vi "Get_ADAM_Ch_names_client.vi"(1 "Channel names set":T1) -> (0 "Ch names":string[](array[string]))   [LabVIEW 2022 SP3]
doc: "This is an example of using features of the VI Server as a client. It shows how you might browse from one or more applications that may be exporting data from one or more data stations. \n\nThe example shows how to query a server for its list of exported VIs, how to get references to the VIs, and how call them with the Call By Reference function."
uses:
  Sub VIs/ADAM Controls/Channel_names.ctl
  Anemometry/Anemometry Sub Vis/Controls/Global_mode.ctl
  Sub VIs/ADAM Controls/Channel_State.ctl
  Anemometry/Anemometry Sub Vis/Globals/Preference_global.vi
panel:
  in  "Server type":refnum<vi>
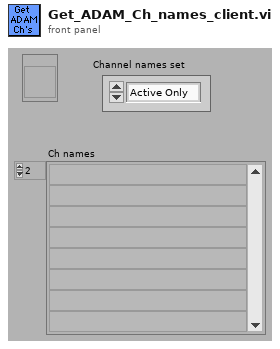
[diagram p1: front panel]
types:
  T1 = typedef "Channel_names.ctl" = enum16{"Active Only", "Active + Off", "All Channels", "Changeable Only", "Always Off", "Always On", "Always Off or On"}
  T2 = typedef "Server_Comms.ctl" = enum16{"Do Not Link To Server", "Server Link Healthy"}
  T3 = typedef "Global_mode.ctl" = enum16{"Read Global", "Load Global From File", "Write Global to File"}
  T4 = typedef "Channel_State.ctl" = enum16{"On", "Off", "Always On", "Always Off"}
  T5 = typedef "Ch_description_ADAM.ctl" = cluster{"Ch Name":string, "Type":T6, "Function":T7, "Ch State":T4, "Calibration type":T8, "A":dbl, "B":dbl, "C":dbl, "D":dbl, "Comments":string, "Address":T9, "String":string, "Duty":u16}
  T6 = typedef "Module_type_ADAM.ctl" = string
  T7 = typedef "Function_ADAM.ctl" = enum16{"Analogue Input", "Digital Input", "Event counter", "Event rate", "Analogue Output", "Digital Output", "Relay Output"}
  T8 = typedef "Calib_type_ADAM.ctl" = string
  T9 = typedef "Address.ctl" = cluster{"Main":i32, "Ch.":i32, "Sub":i32, "Port Name":string}
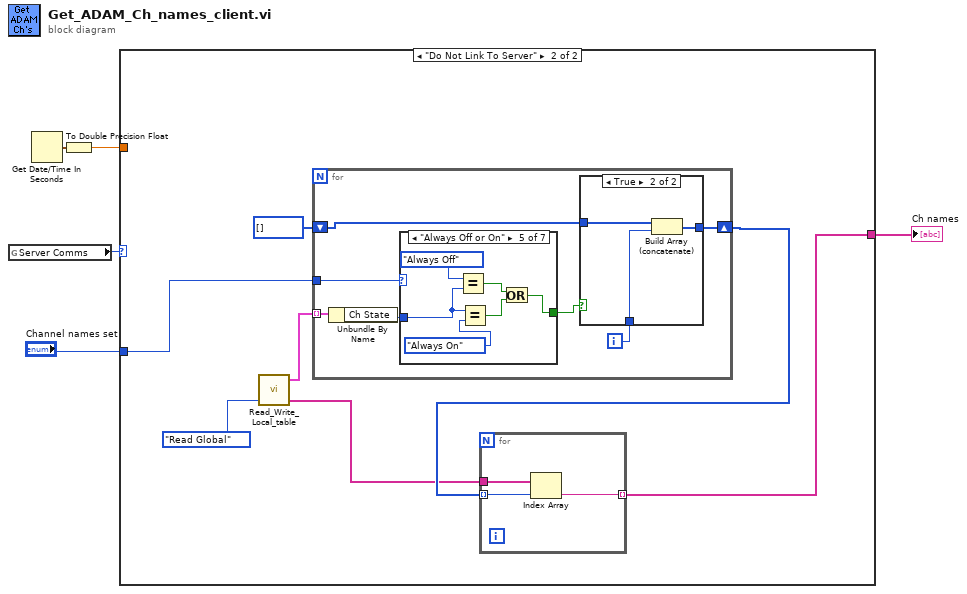
[diagram p0: block diagram]
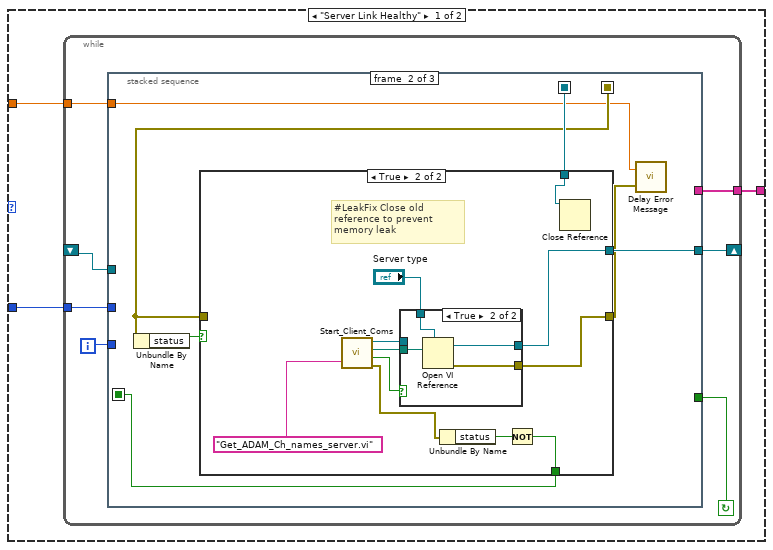
[diagram p2: hidden frame]
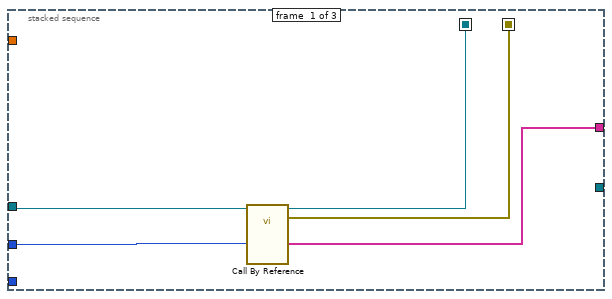
[diagram p3: hidden frame]
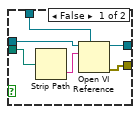
[diagram p5: hidden frame]
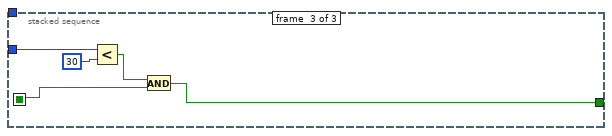
[diagram p6: hidden frame]
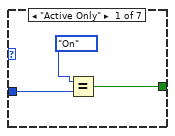
[diagram p8: hidden frame]
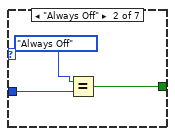
[diagram p9: hidden frame]
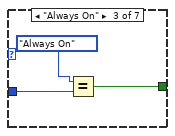
[diagram p10: hidden frame]
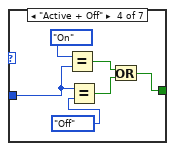
[diagram p11: hidden frame]
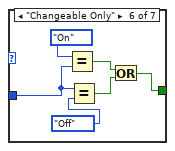
[diagram p12: hidden frame]
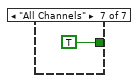
[diagram p13: hidden frame]
diagram:
  n1 = global read "Preference_global.vi" "Server Comms"() -> (w4:T2)
  n2 = Get Date/Time In Seconds() -> (seconds since 1Jan1904=w2:timestamp)
  n3 = To Double Precision Float(number=w2) -> (double precision float=w1:dbl)
  n4 = case shown="\"Do Not Link To Server\"" w4 {
    tunnel: [w8 w57] -> w5
    tunnel: "Channel names set" -> [w7 w61]
    tunnel: w1 -> [w6 _]
    frame "Server Link Healthy" {
      n5 = while {
        tunnel: [w11] -> w8
        shift-left: _ -> [w15]
        shift-right: [w14] -> _
        tunnel: w7 -> [w10]
        tunnel: w6 -> [w9]
        i -> [w13]
        stop <- w12 continue-if-true
        n6 = stacked-sequence {
          seq-local: [w18 _ _] -> [_ w26 _]
          seq-local: [w17 _ _] -> [_ w24 _]
          seq-local: [_ w21 _] -> [_ _ w53]
          tunnel: w15 -> [w20 _ _]
          tunnel: [_ w27 _] -> w14
          tunnel: w13 -> [_ _ w54]
          tunnel: [_ _ w52] -> w12
          tunnel: [w19 _ _] -> w11
          tunnel: w10 -> [w16 _ _]
          tunnel: w9 -> [_ w22 _]
          frame #0 {
            n7 = call-by-ref "?"(reference=w20, "Channel names set"=w16) -> (reference out=w18:refnum<vi>, error out=w17:errorcluster, "Ch names"=w19:string[])  [unwired: 1 in]
          }
          frame #1 {
            n8 = Unbundle By Name(w24) -> ("status"=w25:bool)
            n9 = case shown="True" w25 {
              selector: w25 -> [w28 _]
              tunnel: [w30 w37] -> w27
              tunnel: w26 -> [w30 w34]
              tunnel: [w29 w35] -> w23
              tunnel: w24 -> [w29 _]
              tunnel: [w28 w31] -> w21
              frame False {
              }
              frame True {
                # "#LeakFix Close old reference to prevent memory leak"
                n10 = call "Start_Client_Coms.vi"("VI name to run on server"="Get_ADAM_Ch_names_server.vi") -> ("LabVIEW application reference"=w39:refnum<vi>, "Checked VI name"=w40:path, "Local Call"=w38:bool, "Error cluster"=w32:errorcluster)  [unwired: 1 in]
                n11 = case shown="True" w38 {
                  tunnel: [w44 w51] -> w37
                  tunnel: "Server type" -> [w43 w50]
                  tunnel: w40 -> [w47 w49]
                  tunnel: w39 -> [w42 _]
                  tunnel: [w45 w48] -> w35
                  frame False {
                    n12 = Strip Path(path=w47) -> (name=w46:string)  [unwired: 1 out]
                    n13 = Open VI Reference(type specifier VI Refnum (for type only)=w43, application reference (local)=w42, vi path=w46) -> (vi reference=w44:refnum<vi>, error out=w45:errorcluster)  [unwired: 1 in, 2 out]
                  }
                  frame True {
                    n14 = Open VI Reference(type specifier VI Refnum (for type only)=w50, vi path=w49) -> (vi reference=w51:refnum<vi>, error out=w48:errorcluster)  [unwired: 1 in, 3 out]
                  }
                }
                n15 = Unbundle By Name(w32) -> ("status"=w33:bool)
                n16 = Not(x=w33) -> (.not. x?=w31:bool)
                n17 = Close Reference(reference=w34) -> ()  [unwired: 1 in, 1 out]
              }
            }
            n18 = call "Delay Error Message.vi"("error in (no error)"=w23, "Seconds since 1904"=w22) -> ()  [unwired: 2 in]
          }
          frame #2 {
            n19 = Less?(x=w54, y=30) -> (x < y?=w56:bool)
            n20 = And(x=w56, y=w53) -> (x .and. y?=w52:bool)
          }
        }
      }
    }
    frame "Do Not Link To Server" {
      n21 = call "Read_Write_Local_table.vi"("Mode"=Global_mode."Read Global") -> ("Ch Names"=w58:string[], "Channels Descriptions Out"=w62:T5[])  [unwired: 2 in, 1 out]
      n22 = for {
        tunnel: w62 -> [w73] mode=indexing
        tunnel: w61 -> [w72]
        shift-right: [w68] -> w59
        shift-left: i32[] [] -> [w67]
        i -> [w69]
        n23 = Unbundle By Name(w73) -> ("Ch State"=w71:T4)
        n24 = case shown="\"Always Off or On\"" w72 {
          tunnel: w71 -> [w80 w83 w86 w91 w97 w103 _]
          tunnel: [w78 w81 w84 w87 w93 w99 TRUE] -> w70
          frame "Active Only" {
            n25 = Equal?(x=Channel_State."On" ("Ch State"), y=w80) -> (x = y?=w78:bool)
          }
          frame "Always Off" {
            n26 = Equal?(x=Channel_State."Always Off" ("Ch State"), y=w83) -> (x = y?=w81:bool)
          }
          frame "Always On" {
            n27 = Equal?(x=Channel_State."Always On" ("Ch State"), y=w86) -> (x = y?=w84:bool)
          }
          frame "Active + Off" {
            n28 = Equal?(x=Channel_State."On" ("Ch State"), y=w91) -> (x = y?=w88:bool)
            n29 = Equal?(x=w91, y=Channel_State."Off" ("Ch State")) -> (x = y?=w89:bool)
            n30 = Or(x=w88, y=w89) -> (x .or. y?=w87:bool)
          }
          frame "Always Off or On" {
            n31 = Equal?(x=Channel_State."Always Off" ("Ch State"), y=w97) -> (x = y?=w94:bool)
            n32 = Equal?(x=w97, y=Channel_State."Always On" ("Ch State")) -> (x = y?=w95:bool)
            n33 = Or(x=w94, y=w95) -> (x .or. y?=w93:bool)
          }
          frame "Changeable Only" {
            n34 = Equal?(x=Channel_State."On" ("Ch State"), y=w103) -> (x = y?=w100:bool)
            n35 = Equal?(x=w103, y=Channel_State."Off" ("Ch State")) -> (x = y?=w101:bool)
            n36 = Or(x=w100, y=w101) -> (x .or. y?=w99:bool)
          }
          frame "All Channels" {
          }
        }
        n37 = case shown="True" w70 {
          tunnel: w69 -> [_ w77]
          tunnel: [w74 w76] -> w68
          tunnel: w67 -> [w74 w75]
          frame False {
          }
          frame True {
            n38 = Build Array (concatenate)(w75, w77) -> (w76:i32[])
          }
        }
      }
      n39 = for {
        tunnel: w59 -> [w66] mode=indexing
        tunnel: w58 -> [w65]
        tunnel: [w64] -> w57 mode=indexing
        n40 = Index Array(array=w65, index=w66) -> (element=w64:string)
      }
    }
  }
  "Ch names" <- w5
